vi "簇名称修改.vi"(8 "输入名称":string[](array[string]), 11 "簇引用":refnum<vi>) -> ()   [LabVIEW 2013]
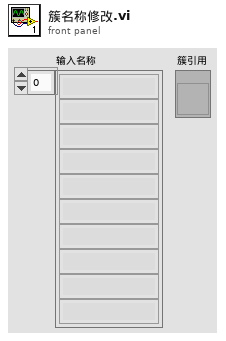
[diagram p1: front panel]
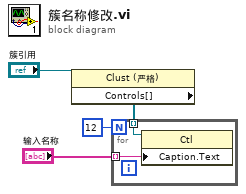
[diagram p0: block diagram]
diagram:
  n1 = property class="Clust (严格)"(reference="簇引用") -> ("Controls[]"=w4:refnum<vi>[])  [unwired: 1 in, 2 out]
  n2 = for {
    N: 12 -> [_]
    tunnel: w4 -> [w6] mode=indexing
    tunnel: "输入名称" -> [w5] mode=indexing
    n3 = property class="Ctl"(reference=w6, "Caption.Text"=w5) -> ()  [unwired: 1 in, 2 out]
  }
